vi "Add LabVIEW Error.vi"(8 "error in (no error)":errorcluster) -> (0 "error out":errorcluster)   [LabVIEW 2015, in "Alarm Handler Actor API.lvclass"]
uses:
  Alarm Handler Actor API.lvclass
  Re-use Libraries/Minimal Actor Framework/Messaging/Message/Message.lvclass/Message.ctl
  <vilib>/GPower/Error/Library/SplitAppended.vi
  <vilib>/GPower/Error/Library/Append/AppendMulti.vi
  <vilib>/GPower/Error/Library/ErrorType.vi
  <vilib>/GPower/Error/Library/SubVIs/ExplanationToError.vi
  <vilib>/dlg_ctls.llb/Space Constant.vi
  Globals.vi
  <vilib>/Utility/error.llb/Trim Whitespace.vi
  <vilib>/Utility/error.llb/Error Code Database.vi
  <vilib>/GPower/Error/Library/SubVIs/HasBuiltInDescription.vi
  <vilib>/GPower/Error/Library/Append/AppendSingle.vi
  Re-use Libraries/Minimal Actor Framework/Messaging/Message/Message.lvclass
  <vilib>/GPower/Error/GPError.lvlib
  Re-use Libraries/Utility/Utility.lvlib
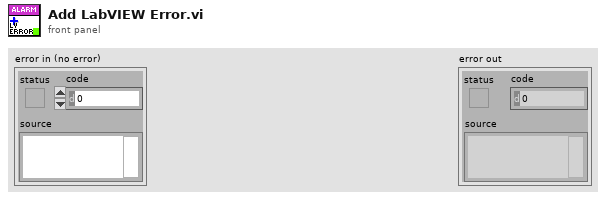
[diagram p1: front panel]
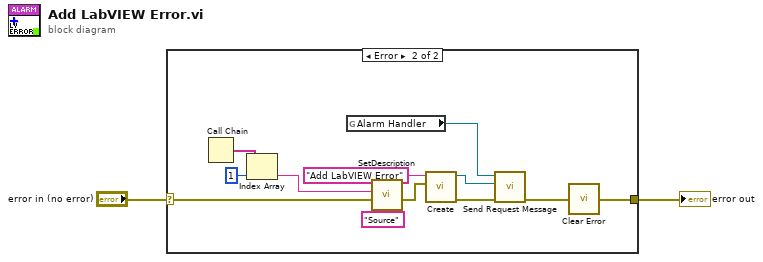
[diagram p0: block diagram]
diagram:
  n1 = case shown="Error" "error in (no error)" {
    selector: "error in (no error)" -> [w3 w7]
    tunnel: [w3 w4] -> w2
    frame No Error {
    }
    frame Error {
      n2 = Call Chain() -> (call chain=w10:string[])
      n3 = Index Array(array=w10, index=1) -> (element=w8:string)
      n4 = global read "Globals.vi" "Alarm Handler"() -> (w11:refnum<class "Alarm Handler Actor API.lvclass">)
      n5 = call <vilib>:"SetDescription.vi"("Label"="Source", "Error in"=w7, "Description"=w8) -> ("Error out"=w6:errorcluster)  [unwired: 8 in]
      n6 = call "Create.vi"("Data"=w6, "Name"="Add LabVIEW Error" ("Parameter")) -> ("error out"=w12:errorcluster, "Message out"=w13:refnum<class "Message.lvclass">)  [unwired: 8 in]
      n7 = call-dynamic "Send Request Message.vi"("error in (no error)"=w12, "Message"=w13, "Actor API in"=w11) -> ("error out"=w15:errorcluster)  [unwired: 8 in]
      n8 = call "Clear Error.vi"("error in (no error)"=w15) -> ("error out"=w4:errorcluster)
    }
  }
  "error out" <- w2
